vi "get object terminals.vi"(8 "error in":errorcluster, 11 "object id":string) -> (0 "error out":errorcluster, 3 "Terminal Description":string)   [LabVIEW 2020]
doc: "Returns the Terminals Names and/or descriptions as a string as well as their Index to be used in other functions like connect objects."
uses:
  G-AI Core/G-AI Core.lvlib
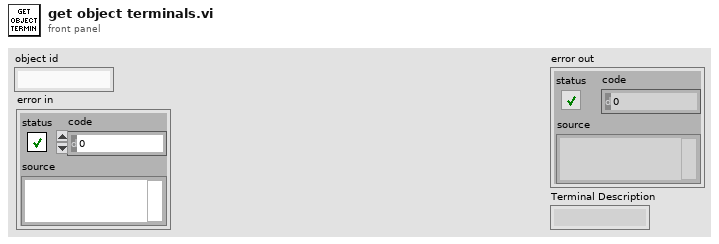
[diagram p1: front panel]
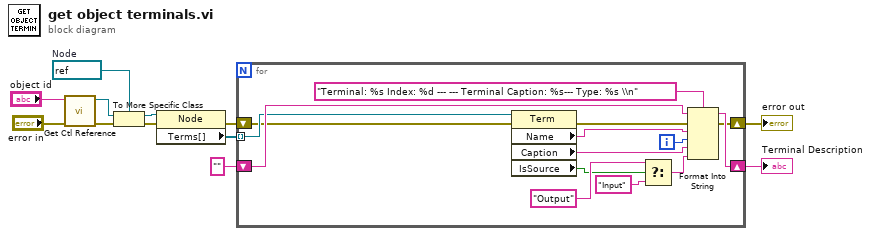
[diagram p0: block diagram]
diagram:
  w9 = refnum<vi> refnum  # Node
  n1 = call "Get Ctl Reference.vi"("error in"="error in", "id"="object id") -> ("error out"=w3:errorcluster, "ctl reference"=w4:refnum<vi>)  [unwired: 8 in]
  n2 = To More Specific Class(target class=w9, reference=w4, error in=w3) -> (specific class reference=w8:refnum<vi>, error out=w7:errorcluster)
  n3 = property class="Node"(reference=w8, error in=w7) -> (error out=w12:errorcluster, "Terms[]"=w11:refnum<vi>[])  [unwired: 1 out]
  n4 = for {
    shift-right: [w25] -> w5
    shift-left: "" -> [w26]
    tunnel: w11 -> [w23] mode=indexing
    shift-right: [w13] -> w6
    shift-left: w12 -> [w22]
    i -> [w15]
    n5 = property class="Term"(reference=w23, error in=w22) -> (error out=w14:errorcluster, "Name"=w17:string, "Caption"=w16:string, "IsSource"=w20:bool)  [unwired: 1 out]
    n6 = Select(t="Output" ("input 4"), s=w20, f="Input" ("input 4")) -> (s? t:f=w19:string)
    n7 = Format Into String(format string="Terminal: %s Index: %d --- --- Terminal Caption: %s--- Type: %s \\n", initial string=w26, error in=w14, w17, w15, w16, w19) -> (resulting string=w25:string, error out=w13:errorcluster)
  }
  "error out" <- w6
  "Terminal Description" <- w5
